vi "dequeue.vi"(8 "error in (no error)":errorcluster, 11 "EventDaemon in":refnum<class "ErrorDaemon.lvclass">) -> (0 "error out":errorcluster, 2 "state":T1, 3 "EventDaemon out":refnum<class "ErrorDaemon.lvclass">, 5 "timeout":i32)   [LabVIEW 2020, in "ErrorDaemon.lvclass"]
doc: "Dequeues private states for daemon."
uses:
  ErrorDaemon.lvclass
  states--enum.ctl
  ErrorDaemon.lvclass/ErrorDaemon.ctl
panel:
  out "data":errorcluster
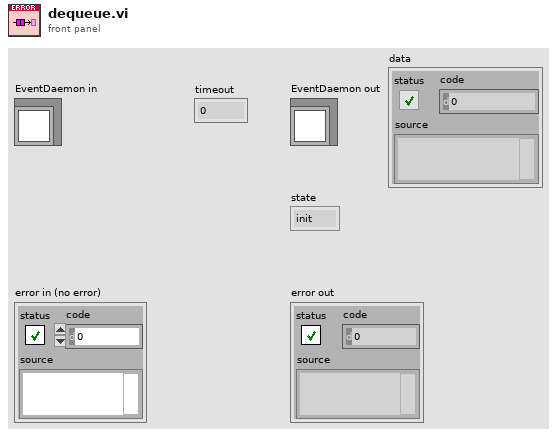
[diagram p1: front panel]
types:
  T1 = typedef "ErrorDaemon.lvclass/states--enum.ctl" = enum16{"init", "default", "display error", "error handler", "exit"}
  T2 = typedef "ErrorDaemon.lvclass/msg--cluster.ctl" = cluster{"cmd":T1, "error":errorcluster}
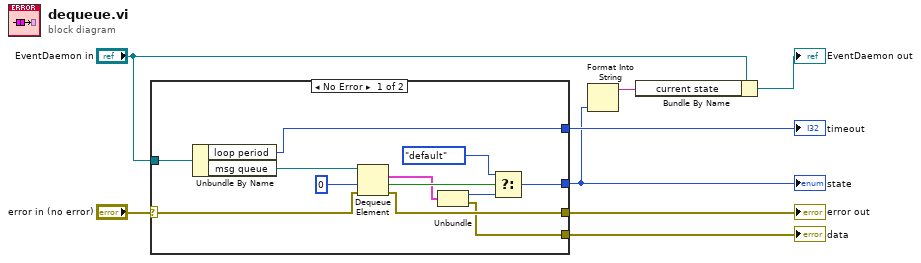
[diagram p0: block diagram]
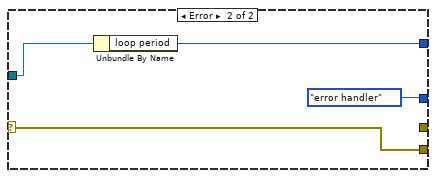
[diagram p2: hidden frame]
diagram:
  n1 = case shown="No Error" "error in (no error)" {
    selector: "error in (no error)" -> [w13 w21]
    tunnel: "EventDaemon in" -> [w20 w23]
    tunnel: [w17 _] -> w8
    tunnel: [w14 states--enum."error handler" ("states")] -> w1
    tunnel: [w12 w22] -> w6
    tunnel: [w9 w21] -> w3
    frame No Error {
      n2 = Unbundle By Name(w20) -> ("loop period"=w12:i32, "msg queue"=w19:refnum<queue>)
      n3 = Dequeue Element(queue=w19, timeout in ms (-1)=0, error in (no error)=w13) -> (element=w11:T2, timed out?=w16:bool, error out=w17:errorcluster)  [unwired: 1 out]
      n4 = Unbundle(w11) -> ("cmd"=w10:T1, "error"=w9:errorcluster)
      n5 = Select(t=states--enum."default", s=w16, f=w10) -> (s? t:f=w14:T1)
    }
    frame Error {
      n6 = Unbundle By Name(w23) -> ("loop period"=w22:i32)
    }
  }
  "error out" <- w8
  "state" <- w1
  "timeout" <- w6
  "data" <- w3
  n7 = Format Into String(w1) -> (resulting string=w2:string)  [unwired: 3 in, 1 out]
  n8 = Bundle By Name(cluster="EventDaemon in", "current state"=w2) -> (→"EventDaemon out":refnum<class "ErrorDaemon.lvclass">)
